vi "Chassis_Sensors.vi"() -> ()   [LabVIEW 2018]
uses:
  Global Variables.vi
  <resource>/objmgr/daqmx.rc
panel:
  out "SubVi Info":T1(array[cluster])
  in  "?":T2={"task/channels in"="MyVoltageTask", "Sample Rate"=1000.0, "samples per channel"=100}
  in  "?":T2={"task/channels in"="MyCurrentTask", "Sample Rate"=1000.0, "samples per channel"=100}
  in  "?":T2={"task/channels in"="TC1", "Sample Rate"=90.0, "samples per channel"=9}
  in  "Alicat_O2":T3={"AR [ B-19200-COM8]"={" ID"="A", "Baud "=enum."19200", "VISA Sesssion In"="COM17"}, "Fluid"="O2"}
  in  "Alicat_Ar":T3={"AR [ B-19200-COM8]"={" ID"="B", "Baud "=enum."19200", "VISA Sesssion In"="COM14"}, "Fluid"="O2"}
  in  "Use Sensor?":bool
  in  "Use Sensor?":bool
  in  "Use Sensor?":bool
  in  "Use Sensor?":bool
  in  "Use Sensor?":bool
  in  "Ring":u16(ring)=1 items=["Alicat", "DAQmx"]
  in  "stop":bool
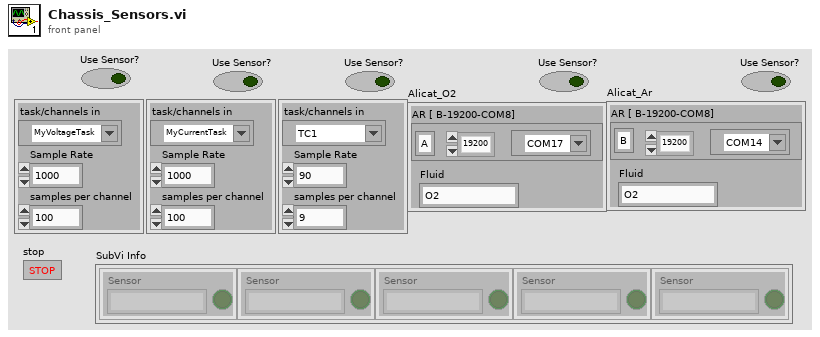
[diagram p1: front panel]
types:
  T1 = cluster{"Sensor":string, "Panel Ref Out":refnum<vi>, bool}[]
  T2 = cluster{"task/channels in":refnum<k21>, "Sample Rate":dbl, "samples per channel":i32}
  T3 = cluster{"AR [ B-19200-COM8]":cluster{" ID":string, "Baud ":enum8{"2400", "9600", "19200", "38400", "57600", "115200", "Unknown"}, "VISA Sesssion In":refnum<visa-resource-name>}, "Fluid":string}
  T4 = enum32{"Invalid", "Standard", "Closed", "Hidden", "Minimized", "Maximized"}
  T5 = cluster{"type":string, "Panel Ref Out":refnum<vi>, bool}
  T6 = enum32{"Bad", "Idle", "Run top level", "Running"}
  T7 = cluster{"task/channels in":string, "Panel Ref Out":refnum<vi>, bool}[]
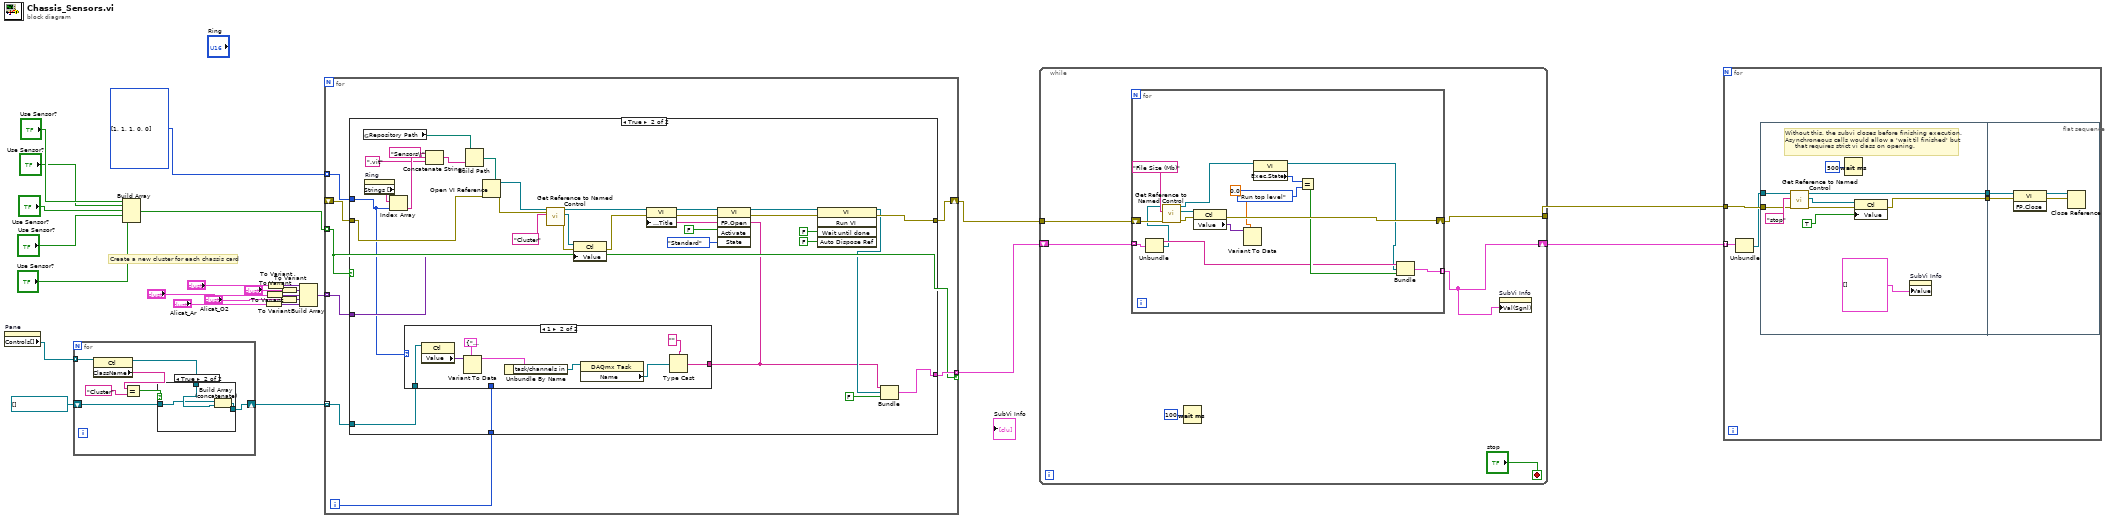
[diagram p0: block diagram]
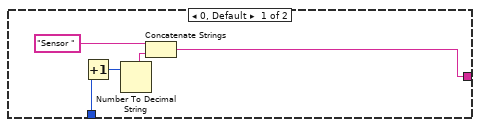
[diagram p4: hidden frame]
diagram:
  w13 = u16[] [1, 1, 1, 0, 0] items=["Alicat", "DAQmx"] ("Array 2")
  # "Create a new cluster for each chassis card"
  n1 = property on="Pane" class="Pane"() -> ("Controls[]"=w11:refnum<vi>[])  [unwired: 2 in, 2 out]
  n2 = for {
    tunnel: w11 -> [w32] mode=indexing
    shift-right: [w27] -> w9
    shift-left: refnum<vi>[] [] -> [w26]
    n3 = property class="Ctl"(reference=w32) -> (reference out=w28:refnum<vi>, "ClassName"=w29:string)  [unwired: 1 in, 1 out]
    n4 = Equal?(x=w29, y="Cluster") -> (x = y?=w31:bool)
    n5 = case shown="True" w31 {
      tunnel: w28 -> [_ w35]
      tunnel: [w33 w36] -> w27
      tunnel: w26 -> [w33 w34]
      frame False {
      }
      frame True {
        n6 = Build Array (concatenate)(w34, w35) -> (w36:refnum<vi>[])
      }
    }
  }
  n7 = Build Array("Use Sensor?", "Use Sensor?", "Use Sensor?", "Use Sensor?", "Use Sensor?") -> (w3:bool[])
  n8 = To Variant(anything="Alicat_Ar") -> (Variant=w14:variant)
  n9 = To Variant(anything="?") -> (Variant=w16:variant)
  n10 = To Variant(anything="?") -> (Variant=w18:variant)
  n11 = To Variant(anything="Alicat_O2") -> (Variant=w15:variant)
  n12 = To Variant(anything="?") -> (Variant=w17:variant)
  n13 = Build Array(w18, w17, w16, w15, w14) -> (w12:variant[])
  n14 = for {
    tunnel: w13 -> [w43] mode=indexing
    tunnel: w12 -> [w42] mode=indexing
    tunnel: w9 -> [w40] mode=indexing
    tunnel: w3 -> [w38] mode=indexing
    shift-right: [w44] -> w25
    shift-left: _ -> [w39]
    tunnel: [w41] -> w2 mode=indexing if=w38
    i -> [w37]
    n15 = case shown="True" w38 {
      tunnel: [w45 w68] -> w44
      tunnel: w43 -> [_ w54]
      tunnel: w42 -> [_ w60]
      tunnel: [_ w56] -> w41
      tunnel: w40 -> [_ w55]
      tunnel: w39 -> [w45 w58]
      tunnel: w37 -> [_ w53]
      frame False {
      }
      frame True {
        n16 = global read "Global Variables.vi" "Repository Path"() -> (w76:path)
        n17 = property on="Ring" class="Ring (strict)"() -> ("Strings []"=w65:string[])  [unwired: 2 in, 2 out]
        n18 = Index Array(array=w65, index=w54) -> (element=w62:string)
        n19 = case shown="1" w54 {
          tunnel: w55 -> [_ w85]
          tunnel: [w79 w83] -> w46
          tunnel: w53 -> [w82 _]
          frame 0, Default {
            n20 = Increment(x=w82) -> (x+1=w78:i32)
            n21 = Number To Decimal String(number=w78) -> (decimal integer string=w80:string)  [unwired: 1 in]
            n22 = Concatenate Strings("Sensor ", w80) -> (w79:string)
          }
          frame 1 {
            n23 = property class="Ctl"(reference=w85) -> ("Value"=w90:variant)  [unwired: 1 in, 2 out]
            n24 = Variant To Data(type=T2 {"task/channels in"="TC1", "Sample Rate"=90.0, "samples per channel"=9} ("PXI-4353 2"), Variant=w90) -> (data=w88:T2)  [unwired: 1 in, 1 out]
            n25 = Unbundle By Name(w88) -> ("task/channels in"=w84:refnum<k21>)
            n26 = property class="DAQmx Task"(reference=w84) -> ("Name"=w87:refnum<k21>)  [unwired: 1 in, 2 out]
            n27 = Type Cast(type="", x=w87) -> (*(type *) &x=w83:string)
          }
        }
        n28 = Concatenate Strings("Sensors\\" ("string"), w62, ".vit" ("string")) -> (w64:string)
        n29 = Build Path(base path=w76, name or relative path=w64) -> (appended path=w77:path)
        n30 = Open VI Reference(vi path=w77, error in (no error)=w58) -> (vi reference=w70:refnum<vi>, error out=w69:errorcluster)  [unwired: 4 in]
        n31 = call "Get Reference to Named Control.vi"("error in (no error)"=w69, "Control Name"="Cluster" ("element"), "Front Panel Ref"=w70) -> ("error out"=w73:errorcluster, "Ctl Refnum"=w74:refnum<vi>, "Panel Ref Out"=w52:refnum<vi>)  [unwired: 6 in]
        n32 = property class="Ctl"(reference=w74, error in=w73, "Value"=w60) -> (error out=w50:errorcluster)  [unwired: 1 out]
        n33 = property class="VI"(reference=w52, error in=w50, "Front Panel.Title"=w46) -> (reference out=w51:refnum<vi>, error out=w49:errorcluster)
        n34 = invoke class="VI" method="FP.Open"(reference=w51, error in=w49, "Activate"=FALSE ("Wait Until Done"), "State"=T4."Standard") -> (reference out=w47:refnum<vi>, error out=w48:errorcluster)  [unwired: 1 in, 3 out]
        n35 = invoke class="VI" method="Run VI"(reference=w47, error in=w48, "Wait until done"=FALSE ("Wait Until Done"), "Auto Dispose Ref"=FALSE ("Auto Dispose Reference")) -> (reference out=w57:refnum<vi>, error out=w68:errorcluster)  [unwired: 1 in, 3 out]
        n36 = Bundle("type"=w46, "Panel Ref Out"=w57, FALSE) -> (w56:T5)  [unwired: 1 in]
      }
    }
  }
  n37 = while {
    tunnel: w25 -> [w96]
    tunnel: [w94] -> w24
    shift-right: [w91] -> w1
    shift-left: w2 -> [w93]
    stop <- "stop" stop-if-true
    n38 = for {
      shift-right: [w110] -> w94
      shift-left: w96 -> [w109]
      tunnel: [w102] -> w91 mode=indexing
      tunnel: w93 -> [w101] mode=indexing
      n39 = Unbundle(w101) -> ("type"=w100:string, "Panel Ref Out"=w99:refnum<vi>)  [unwired: 1 out]
      n40 = call "Get Reference to Named Control.vi"("error in (no error)"=w109, "Control Name"="File Size (Mb)" ("element"), "Front Panel Ref"=w99) -> ("error out"=w108:errorcluster, "Ctl Refnum"=w112:refnum<vi>, "Panel Ref Out"=w98:refnum<vi>)  [unwired: 6 in]
      n41 = property class="Ctl"(reference=w112, error in=w108) -> (error out=w110:errorcluster, "Value"=w107:variant)  [unwired: 1 out]
      n42 = Variant To Data(type=0.0, Variant=w107) -> ()  [unwired: 1 in, 2 out]
      n43 = property class="VI"(reference=w98) -> (reference out=w97:refnum<vi>, "Exec.State"=w105:T6)  [unwired: 1 in, 1 out]
      n44 = Equal?(x=w105, y=T6."Run top level" ("Execution:State 2")) -> (x = y?=w103:bool)
      n45 = Bundle("type"=w100, "Panel Ref Out"=w97, w103) -> (w102:T5)  [unwired: 1 in]
    }
    n46 = Wait (ms)(milliseconds to wait=u32 100) -> ()  [unwired: 1 out]
    n47 = property on="SubVi Info" class="Arr (strict)"("Val(Sgnl)"=w91) -> ()  [unwired: 2 in, 2 out]
  }
  n48 = for {
    tunnel: w24 -> [w117]
    tunnel: w1 -> [w114] mode=indexing
    n49 = Unbundle(w114) -> ("Panel Ref Out"=w113:refnum<vi>)  [unwired: 2 out]
    n50 = flat-sequence {
      tunnel: w117 -> [w125]
      tunnel: [w122] -> w116
      tunnel: [w121] -> w115
      tunnel: w113 -> [w119]
      tunnel: w116 -> [w129]
      tunnel: w115 -> [w128]
      frame #0 {
        # "Without this, the subvi closes before finishing execution.\nAsynchroneous calls would allow a 'wait til finished' but \n     that requires strict vi class on opening."
        n51 = call "Get Reference to Named Control.vi"("error in (no error)"=w125, "Control Name"="stop", "Front Panel Ref"=w119) -> ("error out"=w123:errorcluster, "Ctl Refnum"=w127:refnum<vi>, "Panel Ref Out"=w122:refnum<vi>)  [unwired: 6 in]
        n52 = Wait (ms)(milliseconds to wait=u32 500) -> ()  [unwired: 1 out]
        n53 = property class="Ctl"(reference=w127, error in=w123, "Value"=TRUE) -> (error out=w121:errorcluster)  [unwired: 1 out]
        n54 = property on="SubVi Info" class="Arr (strict)"("Value"=T7 [] ("SubVi Info")) -> ()  [unwired: 2 in, 2 out]
      }
      frame #1 {
        n55 = invoke class="VI" method="FP.Close"(reference=w129, error in=w128) -> (reference out=w131:refnum<vi>, error out=w130:errorcluster)  [unwired: 1 in, 1 out]
        n56 = Close Reference(reference=w131, error in (no error)=w130) -> ()  [unwired: 1 out]
      }
    }
  }
